vi "Data Acquisition.vi"(0 "Index":i32, 1 "采样时钟源":tag="OnboardClock", 2 "采样率":dbl=48000.0, 5 "最大电压":dbl=10.0, 7 "最小电压":dbl=-10.0, 9 "接线端配置":i32(ring)=10083 items=["默认"=-1, "RSE"=10083, "NRSE"=10078, "差分"=10106, "伪差分"=12529], 11 "error in":errorcluster caption="错误输入", 12 "采样模式":i32(ring)=10178 items=["有限采样"=10178, "连续采样"=10123, "硬件定时单点"=12522], 13 "采样数":i32=100) -> (6 "频率":dbl=483.48181062527254, 10 "幅度":dbl caption="检测到的幅值" format="%.2p", 14 "物理通道":tag="Dev1/ai0", 15 "error out":errorcluster caption="错误输出")   [LabVIEW 2015]
uses:
  <vilib>/Utility/error.llb/DialogType.ctl
  <vilib>/DAQmx/read.llb/DAQmx Read (Analog Wfm 1Chan NSamp).vi
  <vilib>/DAQmx/create/channels.llb/DAQmx Create Channel (AI-Voltage-Basic).vi
  <vilib>/DAQmx/configure/timing.llb/DAQmx Timing (Sample Clock).vi
  <vilib>/DAQmx/miscellaneous.llb/DAQmx Fill In Error Info.vi
  <vilib>/measure/matone.llb/Extract Single Tone Information 1 Chan.vi
  <vilib>/measure/mascope.llb/Amplitude and Levels 1 chan.vi
  <vilib>/measure/NI_MAPro.lvlib
panel:
  out "波形图":waveform(dbl)(graph)={"t0"=timestamp(3577334829.178992 s since 1904-01-01), "dt"=2.0833333333333316e-05, "Y"=[0.002432288984326585, -0.13002137242891107, 0.05082881911608649, 0.015168217966368667, -0.08417202809355956, 0.007526660577143417, -0.00011489681208183208, -0.04596424114743332, 0.010073846373551833, 0.010073846373551833, 0.6697949676433317, 0.004979474780735002, 0.002432288984326585, 0.04828163331967808, 0.004979474780735002, 0.007526660577143417, 0.020262589559185498, 0.0686591196909454, 0.007526660577143417, 0.007526660577143417, 0.007526660577143417, 0.002432288984326585, 0.007526660577143417, 0.015168217966368667, 0.010073846373551833, -0.0026620826084902474, 0.002432288984326585, 0.002432288984326585, 0.004979474780735002, 0.010073846373551833, 0.01262103216996025, 0.01262103216996025, 0.007526660577143417, 0.007526660577143417, 0.004979474780735002, 0.007526660577143417, 0.01262103216996025, -0.00775645420130708, 0.007526660577143417, 0.007526660577143417, 0.002432288984326585, 0.002432288984326585, 0.007526660577143417, -0.1045495144648269, 0.010073846373551833, 0.004979474780735002, 0.3335664425174207, 0.002432288984326585, 0.007526660577143417, 0.05847037650531174, 0.015168217966368667, 0.01262103216996025, -0.03322831216539124, 0.010073846373551833, 0.002432288984326585, -0.0026620826084902474, 0.017715403762777082, 0.015168217966368667, 0.03299851854122758, 0.007526660577143417, 0.002432288984326585, 0.007526660577143417, 0.007526660577143417, 0.007526660577143417, 0.015168217966368667, 0.007526660577143417, 0.004979474780735002, 0.002432288984326585, 0.007526660577143417, 0.004979474780735002, 0.015168217966368667, 0.015168217966368667, 0.007526660577143417, 0.010073846373551833, -0.11728544344686898, 0.002432288984326585, 0.015168217966368667, -0.1045495144648269, 0.007526660577143417, 0.010073846373551833, -0.0026620826084902474, 0.002432288984326585, 0.007526660577143417, 0.010073846373551833, 0.015168217966368667, 0.01262103216996025, 0.007526660577143417, 0.002432288984326585, 0.010073846373551833, 0.007526660577143417, 0.015168217966368667, 0.010073846373551833, 0.004979474780735002, 0.007526660577143417, 0.002432288984326585, 0.002432288984326585, 0.007526660577143417, 0.015168217966368667, 0.002432288984326585, -0.0026620826084902474, 0.010073846373551833, -0.09690795707560165, -0.00011489681208183208, 0.007526660577143417, 0.027904146948410747, 0.007526660577143417, 0.010073846373551833, 0.06356474809812858, 0.002432288984326585, 2.9597149986144977, 3.0743383594528764, 0.015168217966368667, 3.071791173656468, 3.071791173656468, 0.007526660577143417, 3.0488665014887926, 3.064149616267243, 0.015168217966368667, 3.0565080588780176, 3.071791173656468, 0.010073846373551833, 3.051413687285201, 3.0666968020636514, 0.007526660577143417, 3.0565080588780176, 3.0794327310456935, 0.010073846373551833, 3.059055244674426, 3.071791173656468, 0.010073846373551833, 3.0616024304708342, 3.076885545249285, 0.01262103216996025, 3.064149616267243, 3.071791173656468, -0.0026620826084902474, 3.0539608730816092, 3.081979916842102, 0.017715403762777082, 3.071791173656468, 3.071791173656468, 0.01262103216996025, 3.051413687285201, 3.0743383594528764, 0.01262103216996025, 3.191508906087664, 3.0666968020636514, 0.007526660577143417, 3.1762257913092133, 3.071791173656468, 0.01262103216996025, 3.0743383594528764, 3.0794327310456935, 0.010073846373551833, 2.9393375122432306, 3.0666968020636514, 0.002432288984326585, 3.064149616267243, 3.0794327310456935, 0.010073846373551833, 3.0666968020636514, 3.0666968020636514, 0.002432288984326585, 3.064149616267243, 3.071791173656468, 0.01262103216996025, 3.0666968020636514, 3.0743383594528764, 0.007526660577143417, 3.0565080588780176, 3.071791173656468, 0.015168217966368667, 3.0692439878600597, 3.071791173656468, 0.007526660577143417, 3.0361305725067504, 3.064149616267243, 0.010073846373551833, 3.0692439878600597, 3.081979916842102, 0.010073846373551833, 3.064149616267243, 3.064149616267243, 0.002432288984326585, 3.0666968020636514, 3.0794327310456935, 0.015168217966368667, 3.0743383594528764, 3.064149616267243, 0.004979474780735002, 3.0743383594528764, 3.0743383594528764, 0.01262103216996025, 3.0794327310456935, 2.8349028945904853, 0.010073846373551833, 3.0666968020636514, 2.9571678128180894, 0.015168217966368667, 3.0692439878600597], "attributes"=variant("NI_ChannelName"=variant(string "Dev1/ai0"), "NI_UnitDescription"=variant(string "Volts"))}
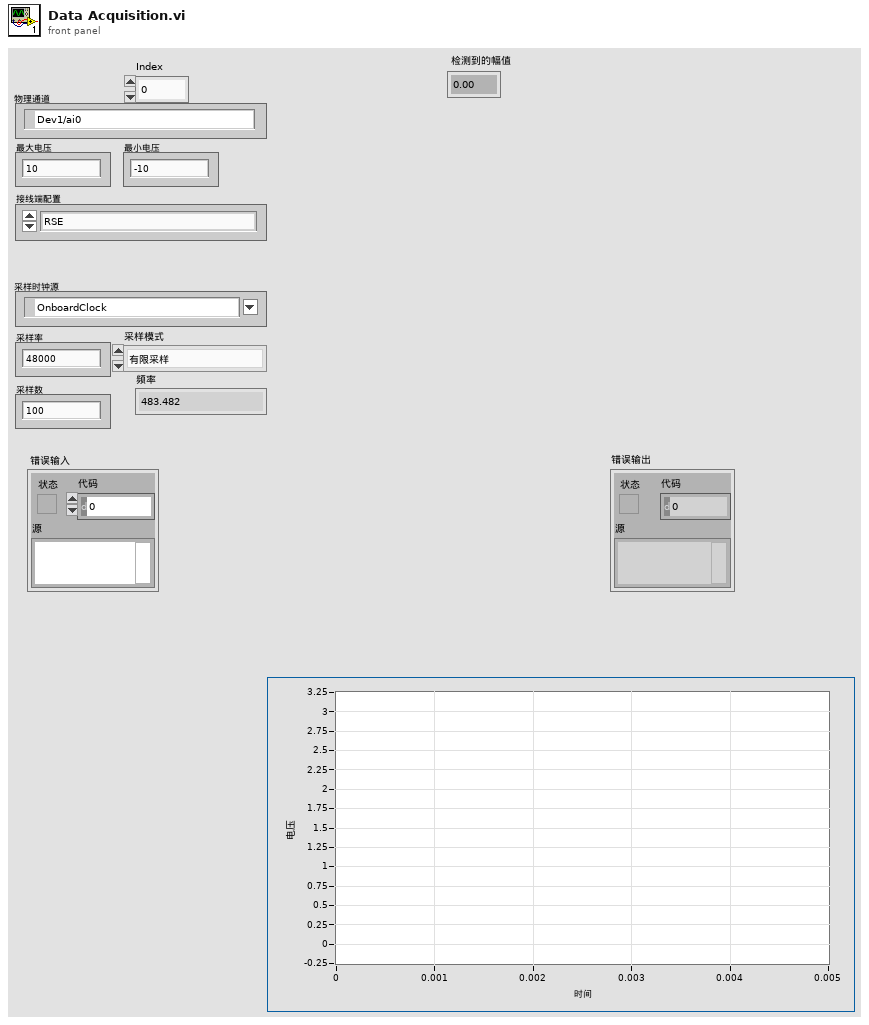
[diagram p1: front panel]
types:
  T1 = typedef "DialogType.ctl" = u16
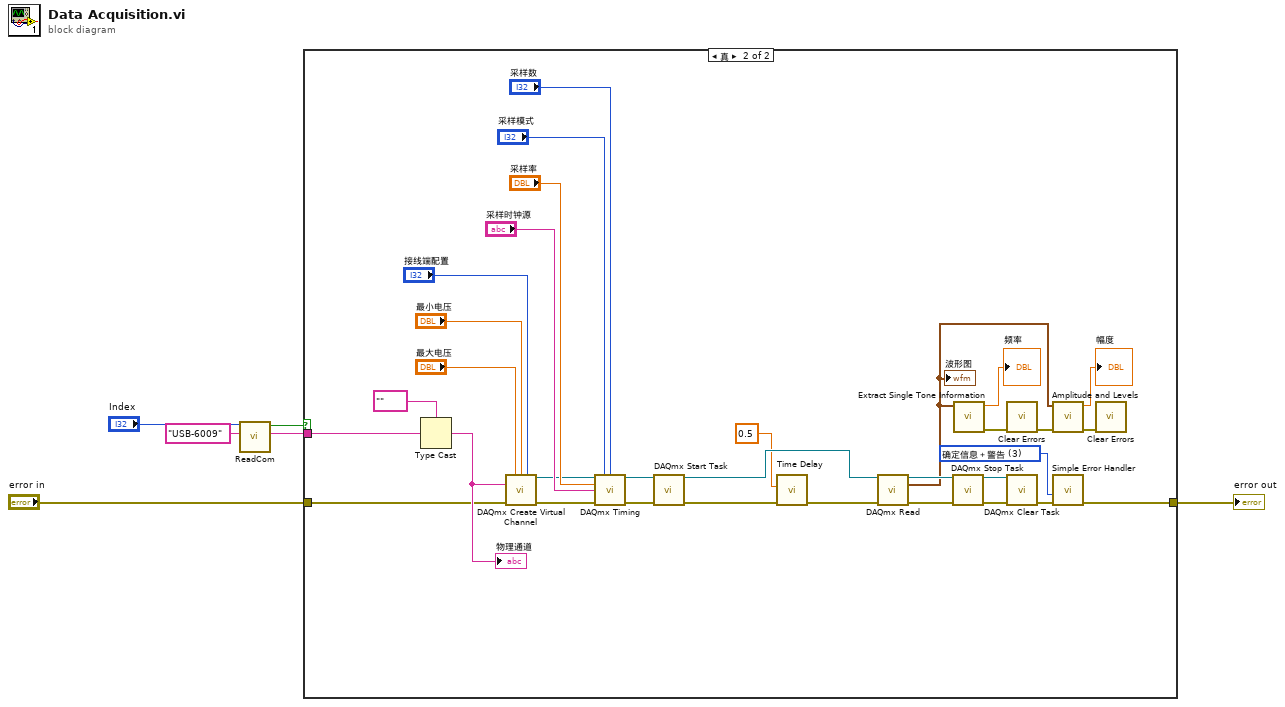
[diagram p0: block diagram]
diagram:
  n1 = call "ReadCom.vi"("仪器名称"="USB-6009", "MyIndex"="Index") -> ("COM"=w1:string, "OK?"=w2:bool)  [unwired: 7 in, 1 out]
  n2 = case shown="真" w2 {
    tunnel: "error in" -> [w7 w17]
    tunnel: [w7 w15] -> w5
    tunnel: w1 -> [_ w8]
    frame False {
    }
    frame True {
      w32 = T1 3 items=["无对话框", "确定信息", "继续或停止信息", "确定信息＋警告", "继续/停止＋警告"] ("对话框类型（确定信息：1）")
      n3 = Type Cast(type=tag "" ("物理通道 2"), x=w8) -> (*(type *) &x=w30:tag)
      "物理通道" <- w30
      n4 = call-poly <vilib>:"DAQmx Create Virtual Channel.vi"("maximum value"="最大电压", "minimum value"="最小电压", "input terminal configuration"="接线端配置", "physical channels"=w30, "error in"=w17) -> ("task out"=w27:refnum<k21>, "error out"=w9:errorcluster)  [unwired: 9 in]
      n5 = call-poly <vilib>:"DAQmx Timing.vi"("task/channels in"=w27, "sample mode"="采样模式", "samples per channel"="采样数", "rate"="采样率", "source"="采样时钟源", "error in"=w9) -> ("task out"=w24:refnum<k21>, "error out"=w10:errorcluster)  [unwired: 8 in]
      n6 = call <vilib>:"DAQmx Start Task.vi"("task/channels in"=w24, "error in"=w10) -> ("task out"=w26:refnum<k21>, "error out"=w11:errorcluster)  [unwired: 12 in]
      n7 = call "Time Delay"("error in (no error)"=w11, "Delay Time (s)"=0.5) -> ("error out"=w23:errorcluster)  [unwired: 9 in]
      n8 = call-poly <vilib>:"DAQmx Read.vi"("task/channels in"=w26, "error in"=w23) -> ("task out"=w25:refnum<k21>, "data"=w18:waveform(dbl), "error out"=w12:errorcluster)  [unwired: 11 in]
      "波形图" <- w18
      n9 = call <vilib>:"DAQmx Stop Task.vi"("task/channels in"=w25, "error in"=w12) -> ("task out"=w20:refnum<k21>, "error out"=w13:errorcluster)  [unwired: 12 in]
      n10 = call-poly <vilib>:"Extract Single Tone Information.vi"("time signal in"=w18) -> ("error out"=w29:errorcluster, "detected frequency"=→"频率":dbl)  [unwired: 5 in, 4 out]
      n11 = call <vilib>:"Clear Errors.vi"("error in (no error)"=w29) -> ("error out"=w19:errorcluster)  [unwired: 5 in, 1 out]
      n12 = call <vilib>:"DAQmx Clear Task.vi"("task in"=w20, "error in"=w13) -> ("error out"=w14:errorcluster)  [unwired: 13 in]
      n13 = call-poly <vilib>:"Amplitude and Levels.vi"("error in (no error)"=w19, "signal in"=w18) -> ("error out"=w21:errorcluster, "amplitude"=→"幅度":dbl)  [unwired: 6 in, 2 out]
      n14 = call <vilib>:"Simple Error Handler.vi"("type of dialog (OK msg:1)"=w32, "error in (no error)"=w14) -> ("error out"=w15:errorcluster)  [unwired: 3 in, 4 out]
      n15 = call <vilib>:"Clear Errors.vi"("error in (no error)"=w21) -> ()  [unwired: 5 in, 2 out]
    }
  }
  "error out" <- w5
